vi "SQL查询.vi"(7 "SQL query":string, 8 "error in (no error)":errorcluster, 11 "database":string) -> (0 "error out":errorcluster, 3 "recordset data":variant[][](array[variant]))   [LabVIEW 2016, in "database.lvlib"]
uses:
  database.lvlib
  <vilib>/Utility/sysdir.llb/System Directory Type.ctl
  <vilib>/addons/database/Connection.llb/DB Tools Open Connec (String).vi
  <vilib>/addons/database/Connection.llb/Conn Execute.vi
  <vilib>/addons/database/Recordset.llb/Rec Fetch Recordset Data (R).vi
  <vilib>/addons/database/Recordset.llb/Rec Destroy - Connection.vi
  <vilib>/addons/database/NI_Database_API.lvlib
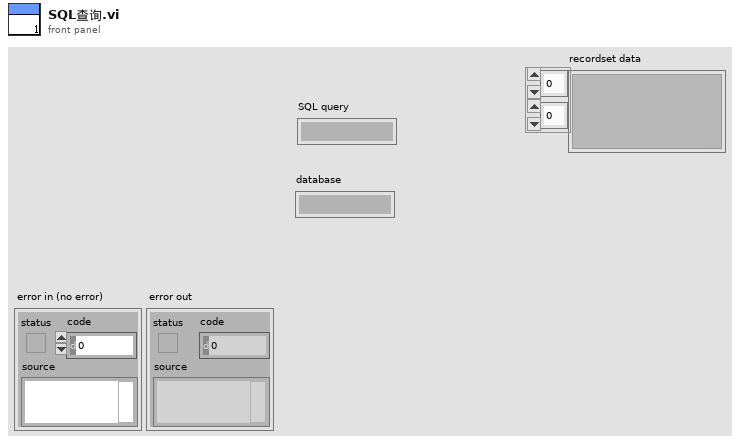
[diagram p1: front panel]
types:
  T1 = typedef "System Directory Type.ctl" = i32
  T2 = typedef "NI_Database_API.lvlib/Conn ObjectReference.ctl" = refnum<k1>
  T3 = typedef "NI_Database_API.lvlib/Rec ObjectReference.ctl" = refnum<k1>
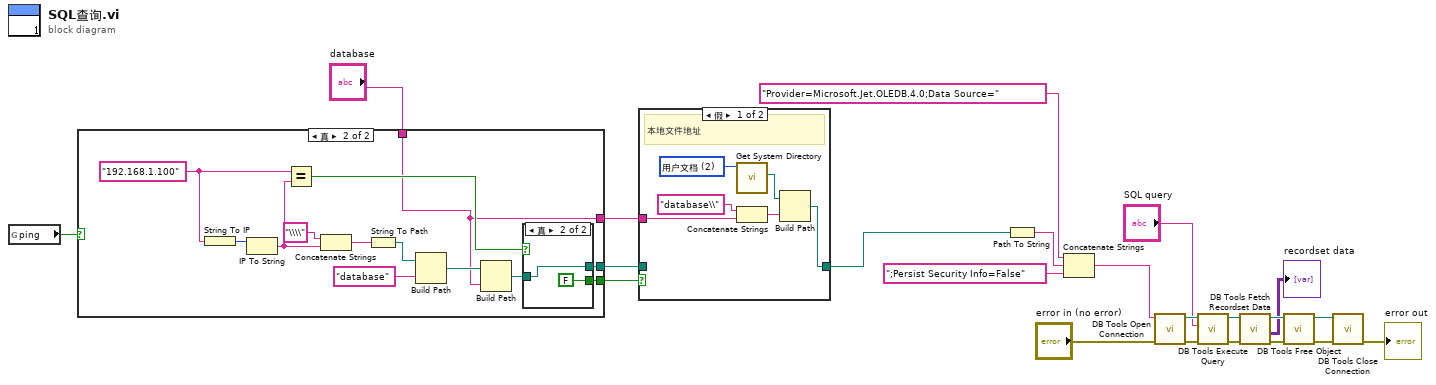
[diagram p0: block diagram]
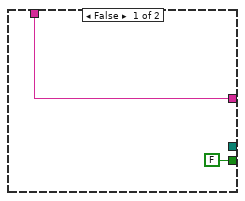
[diagram p2: hidden frame]
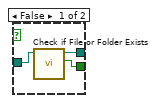
[diagram p3: hidden frame]
diagram:
  n1 = global read "ping全局.vi" "ping"() -> (w3:bool)
  n2 = case shown="真" w3 {
    tunnel: [_ w28] -> w7
    tunnel: [FALSE ("file or folder exists?") w27] -> w6
    tunnel: [w23 w25] -> w4
    tunnel: "database" -> [w23 w25]
    frame False {
    }
    frame True {
      w26 = "192.168.1.100" ("名称")
      n3 = String To IP(1:w26) -> (0:w37:u32)
      n4 = IP To String(2:w37) -> (0:w31:string)  [unwired: 1 in]
      n5 = Equal?(x=w26, y=w31) -> (x = y?=w30:bool)
      n6 = Concatenate Strings("\\\\" ("字符串"), w31) -> (w34:string)
      n7 = String To Path(string=w34) -> (path=w36:path)
      n8 = Build Path(base path=w36, name or relative path="database" ("名称或相对路径")) -> (appended path=w32:path)
      n9 = Build Path(base path=w32, name or relative path=w25) -> (appended path=w29:path)
      n10 = case shown="真" w30 {
        tunnel: w29 -> [w40 w41]
        tunnel: [w39 w41] -> w28
        tunnel: [w38 FALSE] -> w27
        frame False {
          n11 = call <vilib>:"Check if File or Folder Exists.vi"("path"=w40) -> ("file or folder exists?"=w38:bool, "dup path"=w39:path)  [unwired: 8 in, 1 out]
        }
        frame True {
        }
      }
    }
  }
  n12 = case shown="假" w6 {
    tunnel: w4 -> [w44 _]
    tunnel: w7 -> [_ w49]
    tunnel: [w43 w49] -> w5
    frame False {
      w48 = T1 2 items=["用户目录"=0, "用户桌面"=1, "用户文档"=2, "用户应用程序数据"=3, "用户设置"=4, "用户临时目录"=5, "公共文档"=6, "公共应用程序数据"=7, "公共设置"=8, "公共缓存"=13, "系统核心库"=9, "系统安装库"=10, "应用程序文件"=11, "启动盘根目录"=12] ("system directory type")
      # "本地文件地址"
      n13 = call <vilib>:"Get System Directory.vi"("system directory type"=w48) -> ("system directory"=w47:path)  [unwired: 10 in]
      n14 = Concatenate Strings("database\\" ("名称或相对路径"), w44) -> (w45:string)
      n15 = Build Path(base path=w47, name or relative path=w45) -> (appended path=w43:path)
    }
    frame True {
      # "网络共享地址"
    }
  }
  n16 = Path To String(path=w5) -> (string=w8:string)
  n17 = Concatenate Strings("Provider=Microsoft.Jet.OLEDB.4.0;Data Source=", w8, ";Persist Security Info=False") -> (w1:string)
  n18 = call-poly <vilib>:"DB Tools Open Connection.vi"("error in (no error)"="error in (no error)", "connection information"=w1) -> ("error out"=w16:errorcluster, "connection reference"=w17:T2)  [unwired: 6 in]
  n19 = call-poly <vilib>:"DB Tools Execute Query.vi"("error in (no error)"=w16, "SQL query"="SQL query", "connection reference"=w17) -> ("error out"=w15:errorcluster, "recordset reference"=w20:T3)  [unwired: 5 in]
  n20 = call-poly <vilib>:"DB Tools Fetch Recordset Data.vi"("error in (no error)"=w15, "recordset reference"=w20) -> ("error out"=w18:errorcluster, "recordset data"=→"recordset data":variant[][], "recordset reference out"=w19:T3)  [unwired: 3 in]
  n21 = call-poly <vilib>:"DB Tools Free Object.vi"("error in (no error)"=w18, "recordset reference"=w19) -> ("error out"=w13:errorcluster, "connection reference"=w14:T2)  [unwired: 8 in]
  n22 = call <vilib>:"DB Tools Close Connection.vi"("error in (no error)"=w13, "connection reference"=w14) -> ("error out"=→"error out":errorcluster)  [unwired: 5 in]
